vi "Handle Command.vi"(8 "error in (no error)":errorcluster, 9 "Data":variant, 10 "Command":string, 11 "Inst.FP in":refnum<class "Inst.FP.lvclass">) -> (0 "error out":errorcluster, 1 "Processed Data":variant, 2 "Command":string, 3 "Inst.FP out":refnum<class "Inst.FP.lvclass">)   [LabVIEW 2019, in "Inst.FP.lvclass"]
uses:
  Inst.FP.lvclass
  Inst.FP.lvclass/Inst.FP.ctl
  Typedefs/Inst.FP.Get Mode--Cluster.ctl
  Typedefs/Inst.FP.Modes--Enum.ctl
  Typedefs/Inst.FP.getAll--Cluster.ctl
  <userlib>/LevyLab/Instrument Framework/Instrument Types/Cryostat/Instrument.Cryostat.lvclass
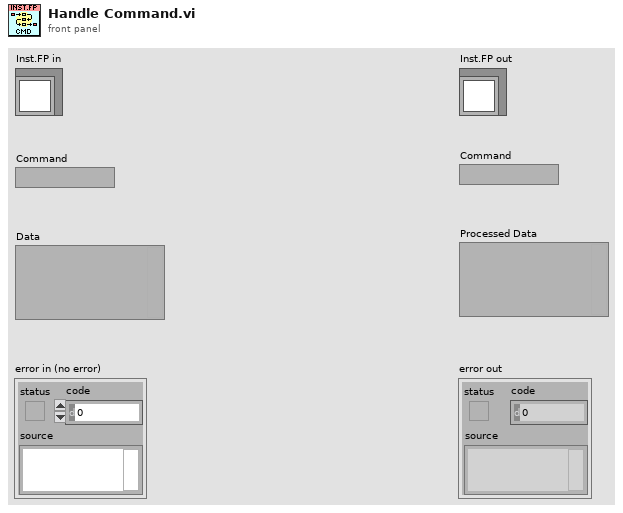
[diagram p1: front panel]
types:
  T1 = typedef "Inst.FP.lvclass/Inst.FP.getAll--Cluster.ctl" = cluster{"FP Data":dbl[], "MG Data":dbl[], "PT Data":dbl[], "Status Array":u32[], "Mode":string}
  T2 = typedef "Inst.FP.lvclass/Inst.FP.Get Mode--Cluster.ctl" = cluster{"Mode":T3}
  T3 = typedef "Inst.FP.lvclass/Inst.FP.Modes--Enum.ctl" = enum16{"AUTO MODE OFF", "START", "CONDENSING 3He", "CONDENSING 4He", "NORMAL CIRCULATION", "RECOVERY OF THE MIXTURE", "RECOVERY: BLOCKAGE or OVERPRESSURE"}
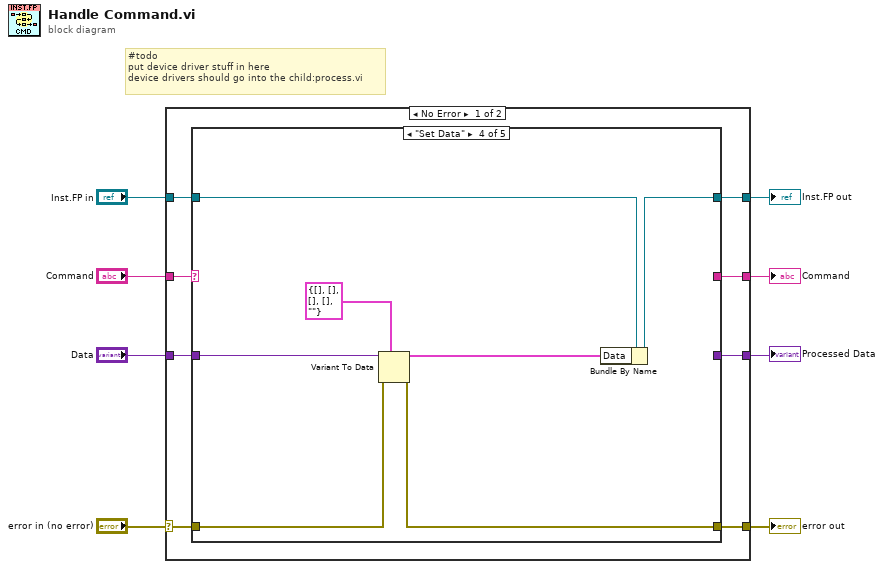
[diagram p0: block diagram]
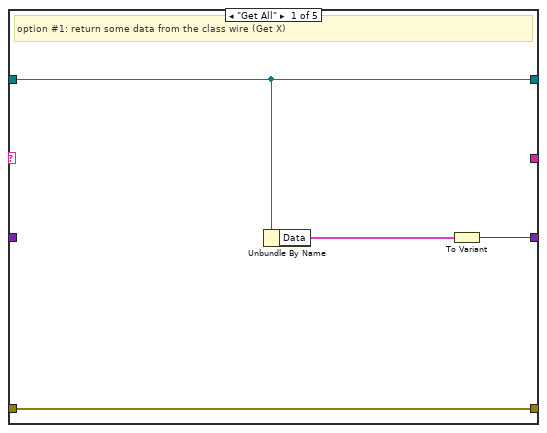
[diagram p2: hidden frame]
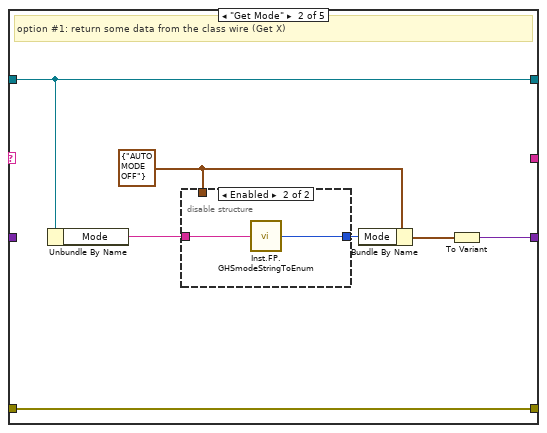
[diagram p3: hidden frame]
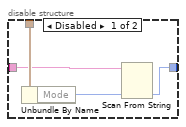
[diagram p4: hidden frame]
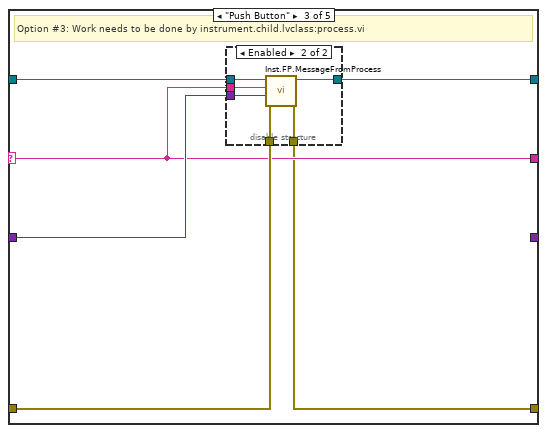
[diagram p5: hidden frame]
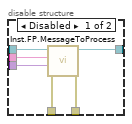
[diagram p6: hidden frame]
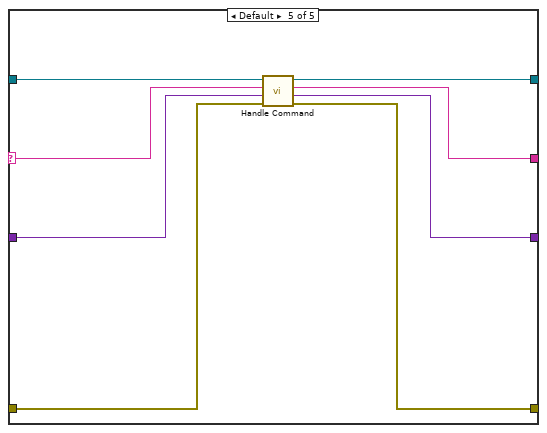
[diagram p7: hidden frame]
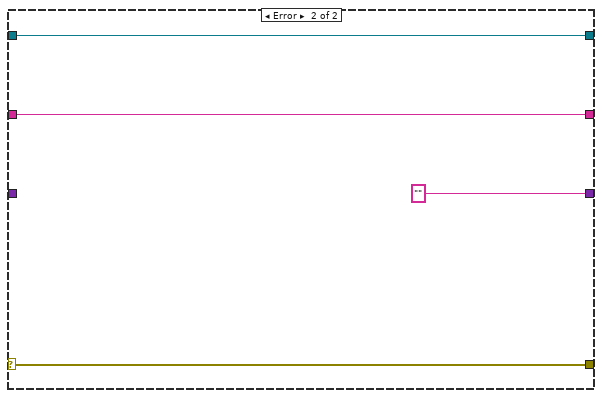
[diagram p8: hidden frame]
diagram:
  # "#todo\nput device driver stuff in here\ndevice drivers should go into the child:process.vi"
  n1 = case shown="No Error" "error in (no error)" {
    selector: "error in (no error)" -> [w10 w70]
    tunnel: [w12 w70] -> w6
    tunnel: [w14 w69] -> w5
    tunnel: "Inst.FP in" -> [w15 w69]
    tunnel: "Command" -> [w16 w67]
    tunnel: [w13 "" ("String")] -> w3
    tunnel: "Data" -> [w9 _]
    tunnel: [w11 w67] -> w1
    frame No Error {
      n2 = case shown="\"Set Data\"" w16 {
        selector: w16 -> [_ _ w36 _ w60]
        tunnel: w15 -> [w19 w27 w39 w58 w64]
        tunnel: [w19 w27 w35 w57 w61] -> w14
        tunnel: [w17 w25 _ _ w63] -> w13
        tunnel: w10 -> [w18 w26 w37 w55 w65]
        tunnel: w9 -> [_ _ w38 w56 w66]
        tunnel: [w18 w26 w34 w54 w62] -> w12
        tunnel: [_ _ w36 _ w59] -> w11
        frame "Get All" {
          # "option #1: return some data from the class wire (Get X)"
          n3 = Unbundle By Name(w19) -> ("Data"=w20:T1)
          n4 = To Variant(anything=w20) -> (Variant=w17:variant)
        }
        frame "Get Mode" {
          w24 = T2 {"Mode"=enum."AUTO MODE OFF"} ("Get Mode")
          # "option #1: return some data from the class wire (Get X)"
          n5 = Unbundle By Name(w27) -> ("Mode"=w21:string)
          n6 = disable-structure shown="Enabled" {
            disable-tunnel: w24 -> [w30 _]
            disable-tunnel: w21 -> [w29 w33]
            disable-tunnel: [w28 w32] -> w22
            frame Disabled {
              n7 = Unbundle By Name(w30) -> ("Mode"=w31:T3)
              n8 = Scan From String(input string=w29, default 1=w31) -> (output 1=w28:T3)  [unwired: 3 in, 3 out]
            }
            frame Enabled {
              n9 = call "Inst.FP.GHSmodeStringToEnum.vi"("mode string"=w33) -> ("mode enum"=w32:T3)
            }
          }
          n10 = Bundle By Name(cluster=w24, "Mode"=w22) -> (w23:T2)
          n11 = To Variant(anything=w23) -> (Variant=w25:variant)
        }
        frame "Push Button" {
          # "Option #3: Work needs to be done by instrument.child.lvclass:process.vi"
          n12 = disable-structure shown="Enabled" {
            disable-tunnel: w39 -> [w45 w51]
            disable-tunnel: w38 -> [w44 w49]
            disable-tunnel: w37 -> [w43 w48]
            disable-tunnel: w36 -> [w42 w50]
            disable-tunnel: [w41 w46] -> w35
            disable-tunnel: [w40 w47] -> w34
            frame Disabled {
              n13 = call "Inst.FP.MessageToProcess.vi"("error in (no error)"=w43, "Data"=w44, "Command"=w42, "Inst.FP in"=w45) -> ("error out"=w40:errorcluster, "Inst.FP out"=w41:refnum<class "Inst.FP.lvclass">)  [unwired: 6 in]
            }
            frame Enabled {
              n14 = call "Inst.FP.MessageFromProcess.vi"("error in (no error)"=w48, "Data"=w49, "Command"=w50, "Inst.FP in"=w51) -> ("error out"=w47:errorcluster, "Inst.FP out"=w46:refnum<class "Inst.FP.lvclass">)  [unwired: 6 in]
            }
          }
        }
        frame "Set Data" {
          n15 = Variant To Data(error in=w55, type=T1 {"FP Data"=[], "MG Data"=[], "PT Data"=[], "Status Array"=[], "Mode"=""} ("getAll"), Variant=w56) -> (data=w53:T1, error out=w54:errorcluster)
          n16 = Bundle By Name(cluster=w58, "Data"=w53) -> (w57:refnum<class "Inst.FP.lvclass">)
        }
        frame Default {
          n17 = call-parent "Handle Command.vi"("error in (no error)"=w65, "Data"=w66, "Command"=w60, "Instrument in"=w64) -> ("error out"=w62:errorcluster, "Processed Data"=w63:variant, "Command"=w59:string, "Instrument out"=w61:refnum<class "Inst.FP.lvclass">)  [unwired: 4 in]
        }
      }
    }
    frame Error {
    }
  }
  "error out" <- w6
  "Inst.FP out" <- w5
  "Command" <- w1
  "Processed Data" <- w3
